vi "trace_display.vi"(0 "Carrier amplitudes":T13 format="%#_3p", 1 "Ref carrier amplitudes":T13 format="%#_3p", 2 "Frequency display":T12, 3 "Spectrogram reference":refnum<vi>, 9 "Config":T19={"IO params"={"Conversion"={"Rate"=4.0, "In cards"=2, "Out channels"=4}, "Carriers"={"Phase shift"=180.0, "Levels"=[[0.8, 0.8, 0.8], [0.03, 0.03, 0.03]], "Delay samples"=73.15}}, "High rate STFT"={"Win param"=101.5, "Window type"=61, "Win order"=2, "DFT size"=64, "Channels"=[7], "Oversample"=64}, "Low rate STFT"={"Win param"=120.0, "Window type"=61, "Win order"=8, "DFT size"=64, "Channels"=[7], "Oversample"=64}, "Filtering"={"Hum"={"Frequency"=0.0, "Tc"=0.0, "Limit"=101.5, "FFT filter"=FALSE, "Detrend mode"=enum."Robust linear", "Enable"=FALSE}, "Kalman"={"Process noise"=101.5, "Measure noise"=101.5}, "Distortion"={"LF cut"=101.5, "Tc"=3.0, "Limit"=101.5, "FFT filter"=FALSE, "Detrend mode"=enum."Robust linear", "Enable"=FALSE}}} {"Filtering"."Distortion"."Limit" format="%#_3p"; "Filtering"."Distortion"."LF cut" format="%#_3p"; "Filtering"."Kalman"."Measure noise" format="%#_3p"; "Filtering"."Kalman"."Process noise" format="%#_3p"; "Filtering"."Hum"."Limit" format="%#_3p"; "Filtering"."Hum"."Frequency" format="%#_4p"; "Low rate STFT"."Oversample" min=1 step=1; "Low rate STFT"."Channels" min=0 step=1; "Low rate STFT"."DFT size" min=1 step=1; "Low rate STFT"."Window type" items=["Rectangle"=0, "Hanning"=1, "Hamming"=2, "Blackman-Harris"=3, "Exact Blackman"=4, "Blackman"=5, "Flat Top"=6, "4 Term B-Harris "=7, "7 Term B-Harris"=8, "Low Sidelobe"=9, "Blackman Nuttall"=11, "Triangle"=30, "Bartlett-Hanning"=31, "Bohman"=32, "Parzen"=33, "Welch"=34, "Kaiser"=60, "Dolph-Chebyshev"=61, "Gaussian"=62]; "High rate STFT"."Oversample" min=1 step=1; "High rate STFT"."Channels" min=0 step=1; "High rate STFT"."DFT size" min=1 step=1; "High rate STFT"."Window type" items=["Rectangle"=0, "Hanning"=1, "Hamming"=2, "Blackman-Harris"=3, "Exact Blackman"=4, "Blackman"=5, "Flat Top"=6, "4 Term B-Harris "=7, "7 Term B-Harris"=8, "Low Sidelobe"=9, "Blackman Nuttall"=11, "Triangle"=30, "Bartlett-Hanning"=31, "Bohman"=32, "Parzen"=33, "Welch"=34, "Kaiser"=60, "Dolph-Chebyshev"=61, "Gaussian"=62]; "IO params"."Carriers"."Levels" min=0.0 step=0.1; "IO params"."Conversion"."Rate" format="%#_8g"}, 10 "Reset":bool, 11 "Modulation info":T18 {"Hi channels at low" min=0 step=1; "Low carriers" format="%#_6p"; "High carriers" format="%#_6p"}, 12 "Display options":T3={"Display card"=0, "Signal"=enum."Raw data", "Source axis"=enum."X", "Sensor axis"=enum."X", "Spectrum parameters"={"Window"=enum."7 Term B-Harris", "FFT blocking"=enum."1", "Averaging"=5.0, "Order"=2}, "AC/DC"=enum."Radio Selection 1", "Levels selectors"=[], "Map selector"=enum."fire", "Restart Averaging"=FALSE, "Noise ref"=FALSE} {"Spectrum parameters"."Order" min=1 max=100; "Spectrum parameters"."Averaging" min=0.0 max=1000.0 step=1.0}, 13 "Trace info":T15) -> (20 "Autocorrelation":T1, 21 "Levels arrays":cluster{"Levels":dbl[][]}[](array[cluster]), 22 "STFT Spectrogram":dbl[][](array[numeric]), 23 "Time domain":waveform(dbl)[](array[waveform]), 24 "Time statistics":T14 {"dB" format="%.1f"; "RMS" format="%#_3p"; "DC" format="%#_3p"; "|max|" format="%#_3p"}, 25 "Spectrum":waveform(dbl)[](array[waveform]), 26 "Noise":T2 {"Noise delta" format="%#_6p"; "Noise floor" format="%#_6p"})   [LabVIEW 2014]
uses:
  ilemt_config.ctl
  IO_params.ctl
  stft_params.ctl
  <vilib>/Analysis/4window.llb/windowTd.ctl
  filter_params.ctl
  detrend_mode.ctl
  modulation_info.ctl
  trace_info.ctl
  trace_channel.ctl
  ilemt_status.ctl
  carrier_amplitudes.ctl
  trace_stats.ctl
  frequency_display_tabs.ctl
  display_options.ctl
  display_source.ctl
  axis_name.ctl
  spectrum_parameters.ctl
  levels_selector.ctl
  Level selector 1.ctl
  Level selector 4.ctl
  Level selector 3.ctl
  Level selector 2.ctl
  <vilib>/Analysis/2dsp.llb/Inverse Real FFT.vi
  <vilib>/Analysis/2dsp.llb/1D Auto Correlation (DBL).vi
  <vilib>/Analysis/NI_AALPro.lvlib
panel:
  in  "Autocorrelation normalization":enum32{"none", "unbiased", "biased"}(ring)=enum."biased"
  # "Options:"
  # "High"
  # "Low"
  # "X"
  # "Y"
  # "Z"
  # "High"
  # "Low"
  # "X"
  # "Y"
  # "Z"
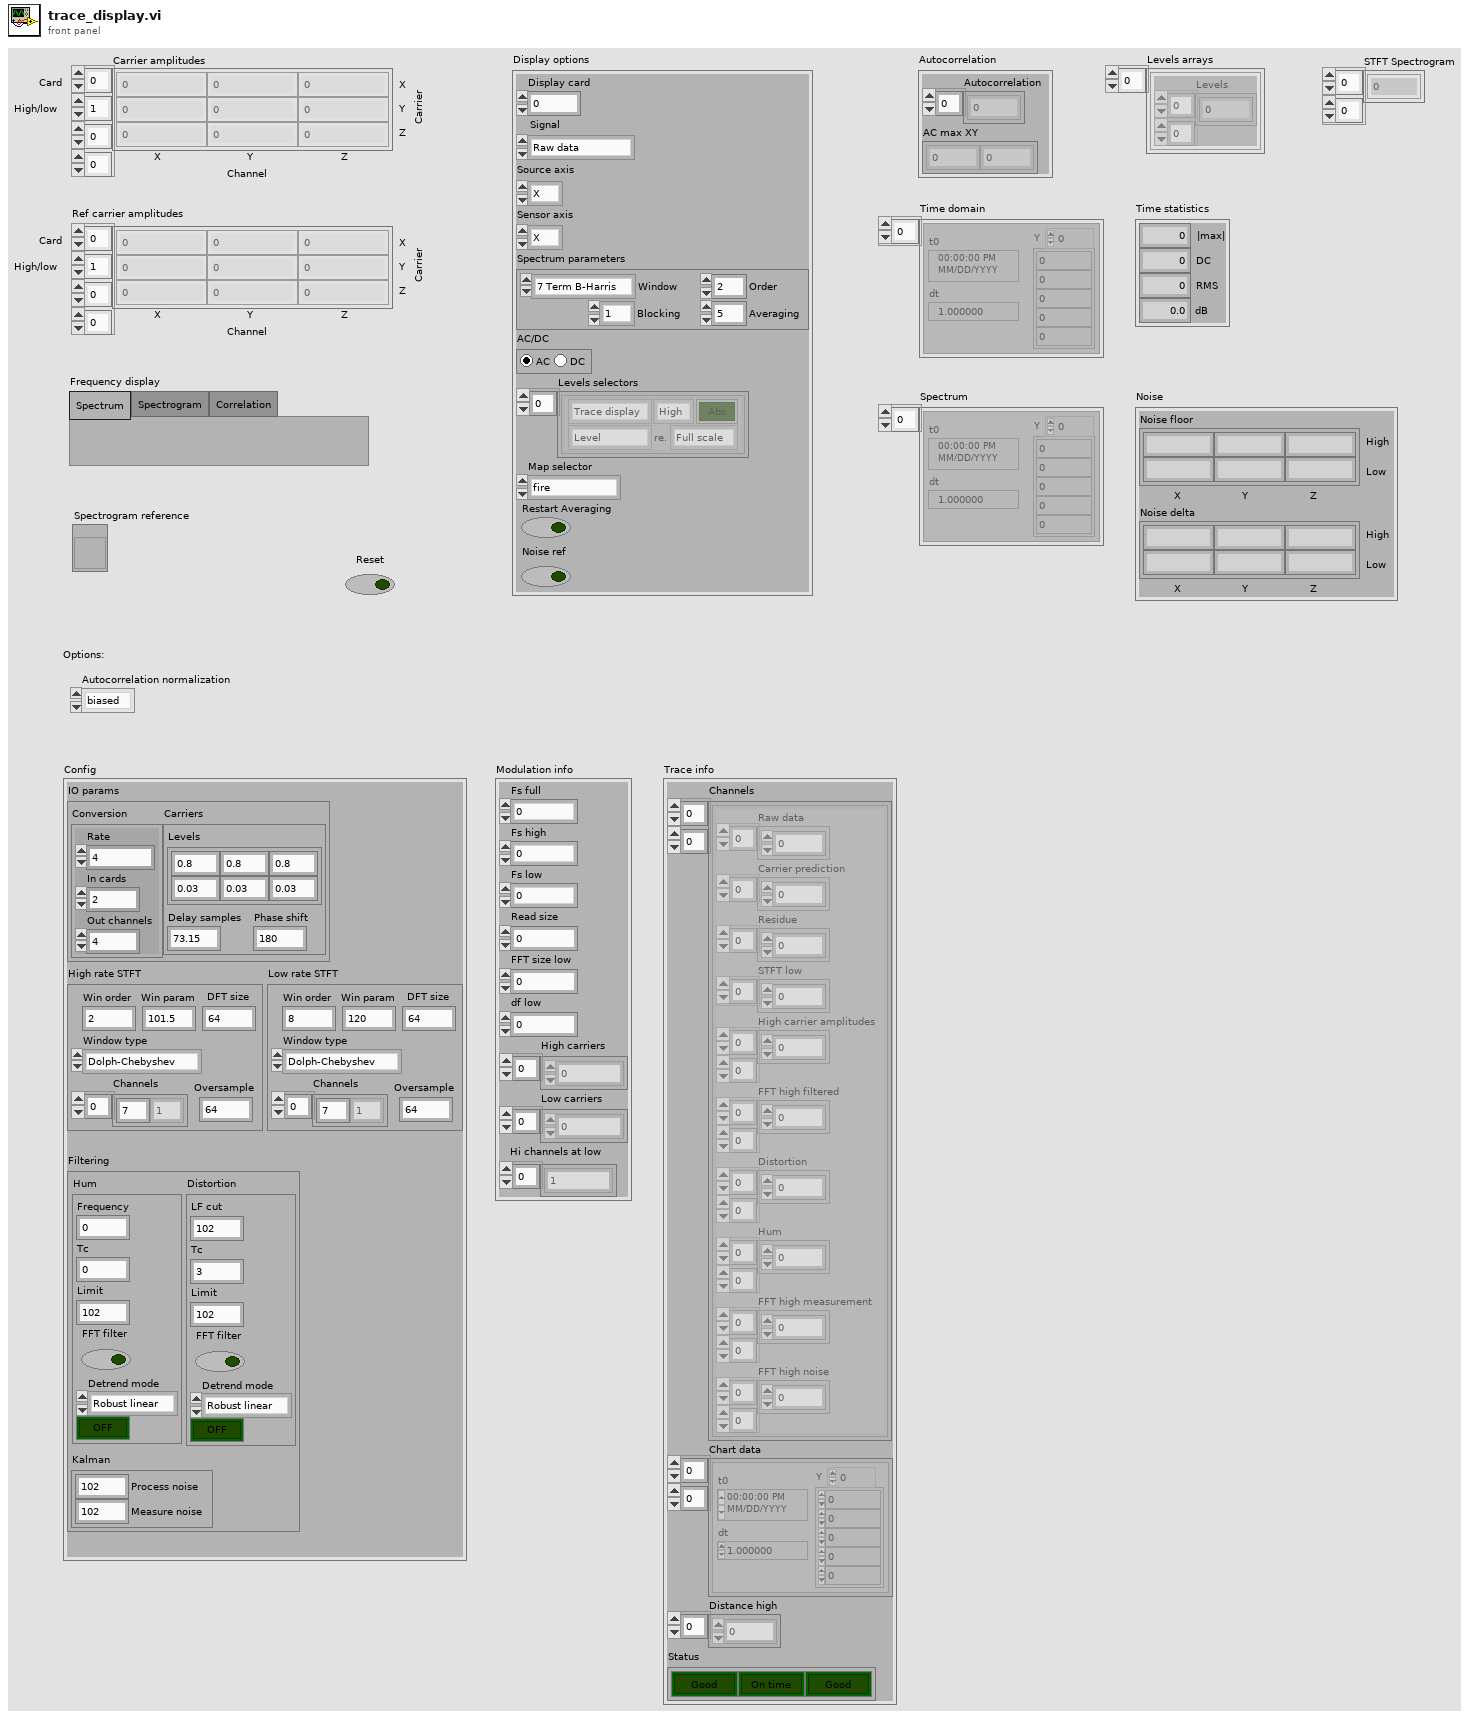
[diagram p1: front panel]
types:
  T1 = cluster{"Autocorrelation":dbl[], "AC max XY":dbl[]}
  T2 = cluster{"Noise floor":dbl[][], "Noise delta":dbl[][]}
  T3 = typedef "display_options.ctl" = cluster{"Display card":i32, "Signal":T4, "Source axis":T5, "Sensor axis":T5, "Spectrum parameters":T6, "AC/DC":enum32{"Radio Selection 1", "Radio Selection 2"}, "Levels selectors":T7[], "Map selector":enum16{"fire", "rainbow", "grey", "inverse grey", "ice", "original"}, "Restart Averaging":bool, "Noise ref":bool}
  T4 = typedef "display_source.ctl" = enum16{"Raw data", "Carrier predict", "Residue", "STFT low", "Hum amplitude", "Hum phase", "Distortion amplitude", "Distortion phase", "FFT high noise", "FFT high measurement", "FFT high filtered", "Amplitude high", "Distance high", "Chart high", "Chart low"}
  T5 = typedef "axis_name.ctl" = enum16{"X", "Y", "Z"}
  T6 = typedef "spectrum_parameters.ctl" = cluster{"Window":enum16{"None ", "Hanning", "Hamming", "Blackman-Harris", "Exact Blackman", "Blackman", "Flat Top", "4 Term B-Harris ", "7 Term B-Harris", "Low Sidelobe"}, "FFT blocking":enum16{"1", "2", "4", "8"}, "Averaging":dbl, "Order":u32}
  T7 = typedef "levels_selector.ctl" = cluster{"Signal source":T8, "Mode":T9, "re.":T10, "High/low":T11, "Sense":bool}
  T8 = typedef "Level selector 1.ctl" = enum16{"Trace display", "Carrier levels", "Ref levels", "Distortion"}
  T9 = typedef "Level selector 4.ctl" = enum16{"Level", "dB", "Phase", "Mismatch"}
  T10 = typedef "Level selector 3.ctl" = enum16{"Full scale", "Carrier", "Ref level", "Noise"}
  T11 = typedef "Level selector 2.ctl" = enum16{"High", "Low"}
  T12 = typedef "frequency_display_tabs.ctl" = enum32{"Spectrum", "Spectrogram", "Correlation"}
  T13 = typedef "carrier_amplitudes.ctl" = cdb[][][][]
  T14 = typedef "trace_stats.ctl" = cluster{"|max|":dbl, "DC":dbl, "RMS":dbl, "dB":dbl}
  T15 = typedef "trace_info.ctl" = cluster{"Channels":T16[][], "Chart data":waveform(dbl)[][], "Distance high":dbl[], "Status":T17}
  T16 = typedef "trace_channel.ctl" = cluster{"Raw data":dbl[], "Carrier prediction":dbl[], "Residue":dbl[], "STFT low":cdb[], "High carrier amplitudes":cdb[][], "FFT high filtered":cdb[][], "Distortion":cdb[][], "Hum":cdb[][], "FFT high measurement":cdb[][], "FFT high noise":dbl[][]}
  T17 = typedef "ilemt_status.ctl" = cluster{"NaN":bool, "Backlog":bool, "Clipping":bool}
  T18 = typedef "modulation_info.ctl" = cluster{"Fs full":dbl, "Fs high":dbl, "Fs low":dbl, "Read size":i32, "FFT size low":i32, "df low":dbl, "High carriers":dbl[], "Low carriers":dbl[], "Hi channels at low":i32[]}
  T19 = typedef "ilemt_config.ctl" = cluster{"IO params":T20, "High rate STFT":T21, "Low rate STFT":T21, "Filtering":T23}
  T20 = typedef "IO_params.ctl" = cluster{"Conversion":cluster{"Rate":dbl, "In cards":u32, "Out channels":u32}, "Carriers":cluster{"Phase shift":dbl, "Levels":dbl[][], "Delay samples":dbl}}
  T21 = typedef "stft_params.ctl" = cluster{"Win param":dbl, "Window type":T22, "Win order":i32, "DFT size":i32, "Channels":i32[], "Oversample":i32}
  T22 = typedef "NI_AALPro.lvlib/windowTd.ctl" = u32
  T23 = typedef "filter_params.ctl" = cluster{"Hum":cluster{"Frequency":dbl, "Tc":dbl, "Limit":dbl, "FFT filter":bool, "Detrend mode":T24, "Enable":bool}, "Kalman":cluster{"Process noise":dbl, "Measure noise":dbl}, "Distortion":cluster{"LF cut":dbl, "Tc":dbl, "Limit":dbl, "FFT filter":bool, "Detrend mode":T24, "Enable":bool}}
  T24 = typedef "detrend_mode.ctl" = enum16{"Zero mean", "Linear", "Robust linear"}
  T25 = enum16{"fire", "rainbow", "grey", "inverse grey", "ice", "original"}
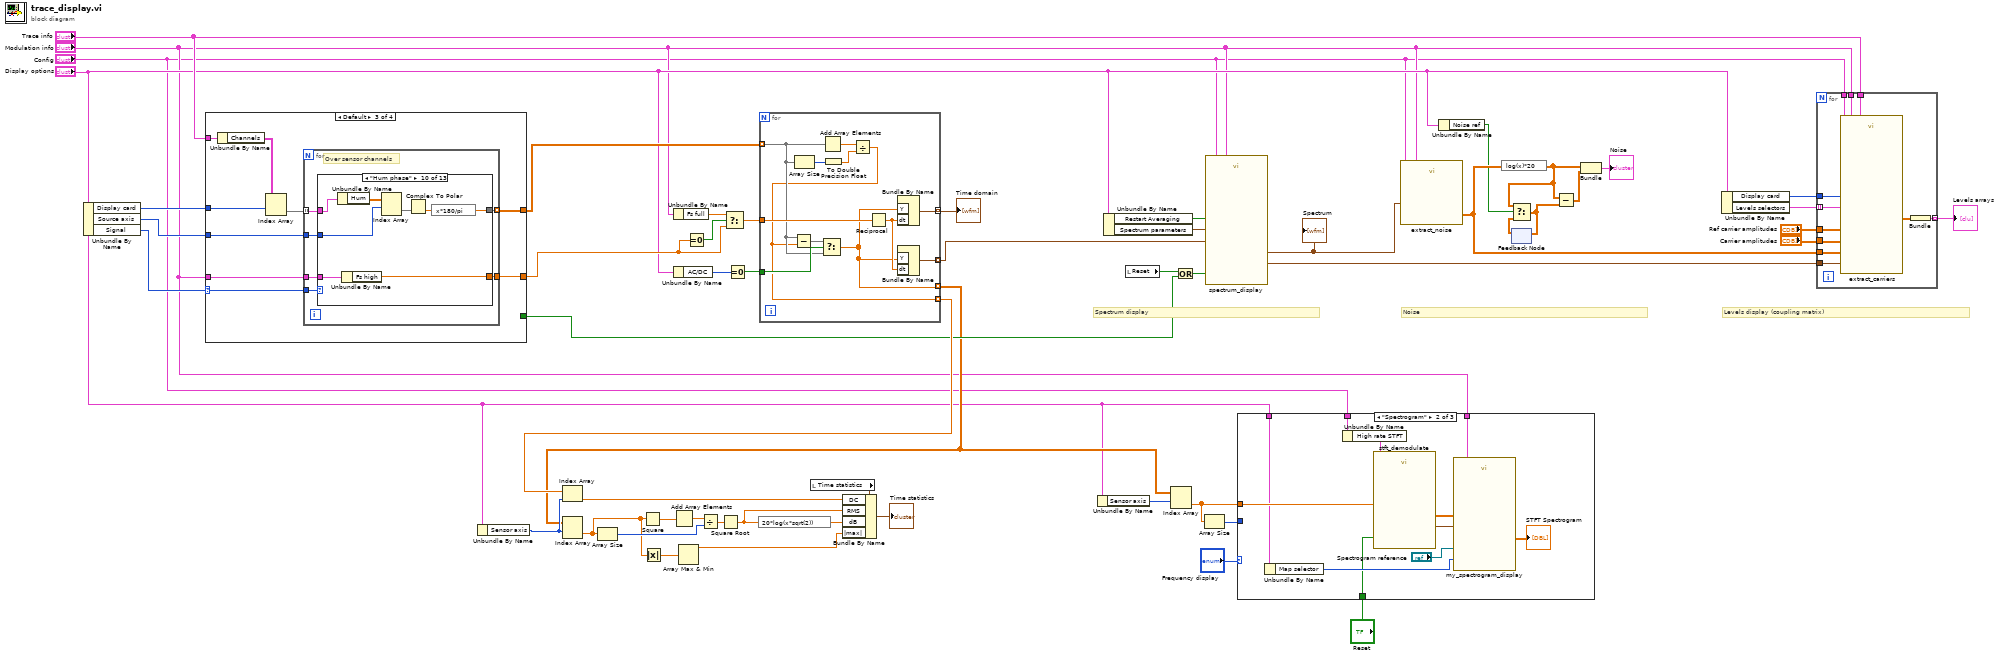
[diagram p0: block diagram]
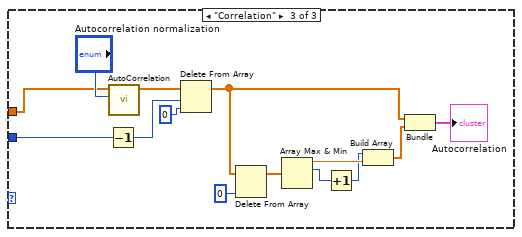
[diagram p3: hidden frame]
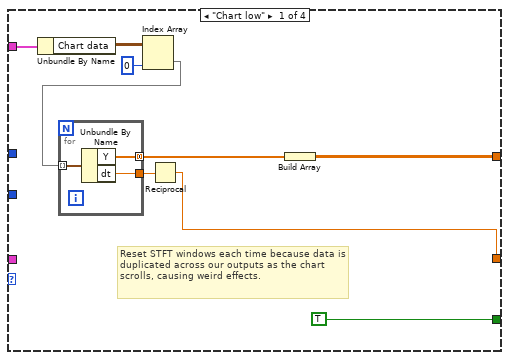
[diagram p4: hidden frame]
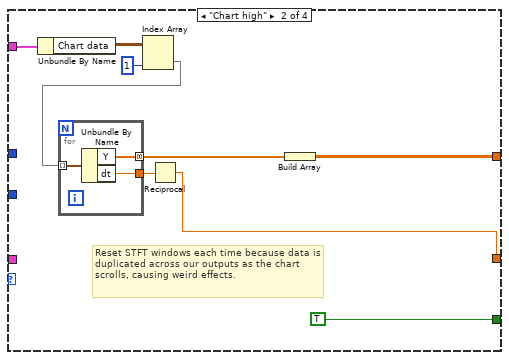
[diagram p5: hidden frame]
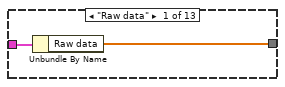
[diagram p6: hidden frame]
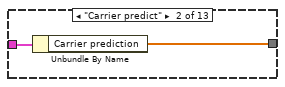
[diagram p7: hidden frame]
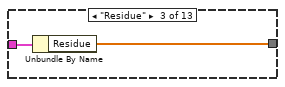
[diagram p8: hidden frame]
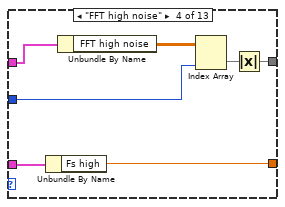
[diagram p9: hidden frame]
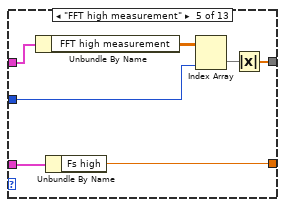
[diagram p10: hidden frame]
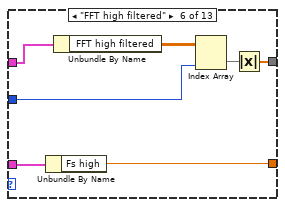
[diagram p11: hidden frame]
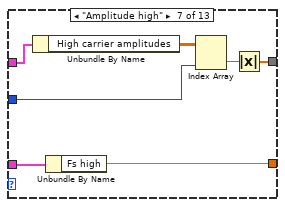
[diagram p12: hidden frame]
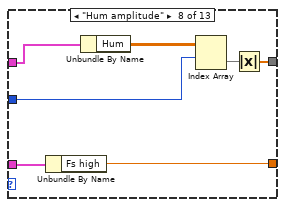
[diagram p13: hidden frame]
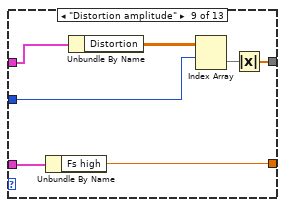
[diagram p14: hidden frame]
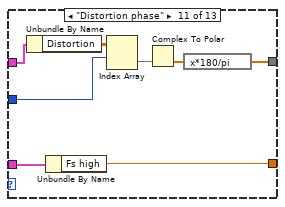
[diagram p15: hidden frame]
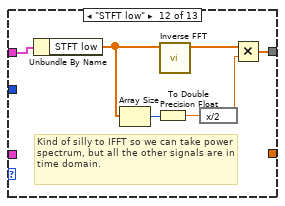
[diagram p16: hidden frame]
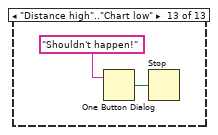
[diagram p17: hidden frame]
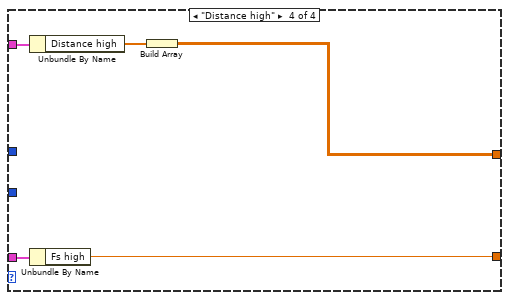
[diagram p18: hidden frame]
diagram:
  # "Levels display (coupling matrix)"
  # "Noise"
  # "Spectrum display"
  n1 = Unbundle By Name("Display options") -> ("Display card"=w25:i32, "Source axis"=w24:T5, "Signal"=w23:T4)
  n2 = case shown="Default" w23 {
    selector: w23 -> [_ _ w84 _]
    tunnel: "Trace info" -> [w60 w72 w85 w170]
    tunnel: [w57 w69 w88 w168] -> w38
    tunnel: "Modulation info" -> [_ _ w87 w172]
    tunnel: [w59 w71 w86 w171] -> w12
    tunnel: [TRUE TRUE _ _] -> w29
    tunnel: w24 -> [_ _ w83 _]
    tunnel: w25 -> [_ _ w80 _]
    frame "Chart low" {
      # "Reset STFT windows each time because data is duplicated across our outputs as the chart scrolls, causing weird effects."
      n3 = Unbundle By Name(w60) -> ("Chart data"=w64:waveform(dbl)[][])
      n4 = Index Array(array=w64, index (col)=0 ("index (row)")) -> (element=w63:waveform(dbl)[])  [unwired: 1 in]
      n5 = for {
        tunnel: w63 -> [w67] mode=indexing
        tunnel: [w66] -> w58 mode=concatenating
        tunnel: [w65] -> w61
        n6 = Unbundle By Name(w67) -> ("Y"=w66:dbl[], "dt"=w65:dbl)
      }
      n7 = Reciprocal(x=w61) -> (1/x=w59:dbl)
      n8 = Build Array(w58) -> (w57:dbl[][])
    }
    frame "Chart high" {
      # "Reset STFT windows each time because data is duplicated across our outputs as the chart scrolls, causing weird effects."
      n9 = Unbundle By Name(w72) -> ("Chart data"=w76:waveform(dbl)[][])
      n10 = Index Array(array=w76, index (col)=1 ("index (row)")) -> (element=w75:waveform(dbl)[])  [unwired: 1 in]
      n11 = for {
        tunnel: w75 -> [w79] mode=indexing
        tunnel: [w78] -> w70 mode=concatenating
        tunnel: [w77] -> w73
        n12 = Unbundle By Name(w79) -> ("Y"=w78:dbl[], "dt"=w77:dbl)
      }
      n13 = Reciprocal(x=w73) -> (1/x=w71:dbl)
      n14 = Build Array(w70) -> (w69:dbl[][])
    }
    frame Default {
      n15 = Unbundle By Name(w85) -> ("Channels"=w82:T16[][])
      n16 = Index Array(array=w82, index (row)=w80) -> (element=w81:T16[])  [unwired: 1 in]
      n17 = for {
        tunnel: [w94] -> w88 mode=indexing
        tunnel: w87 -> [w93]
        tunnel: [w92] -> w86
        tunnel: w84 -> [w91]
        tunnel: w81 -> [w90] mode=indexing
        tunnel: w83 -> [w89]
        # "Over sensor channels"
        n18 = case shown="\"Hum phase\"" w91 {
          tunnel: w90 -> [w96 w98 w100 w107 w114 w121 w128 w135 w142 w150 w158 w165 _]
          tunnel: [w95 w97 w99 w102 w109 w116 w123 w130 w137 w143 w151 w161 _] -> w94
          tunnel: [_ _ _ w105 w112 w119 w126 w133 w140 w148 w156 _ _] -> w92
          tunnel: w93 -> [_ _ _ w106 w113 w120 w127 w134 w141 w149 w157 _ _]
          tunnel: w89 -> [_ _ _ w101 w108 w115 w122 w129 w136 w146 w154 _ _]
          frame "Raw data" {
            n19 = Unbundle By Name(w96) -> ("Raw data"=w95:dbl[])
          }
          frame "Carrier predict" {
            n20 = Unbundle By Name(w98) -> ("Carrier prediction"=w97:dbl[])
          }
          frame "Residue" {
            n21 = Unbundle By Name(w100) -> ("Residue"=w99:dbl[])
          }
          frame "FFT high noise" {
            n22 = Unbundle By Name(w106) -> ("Fs high"=w105:dbl)
            n23 = Unbundle By Name(w107) -> ("FFT high noise"=w104:dbl[][])
            n24 = Index Array(array=w104, index (col)=w101) -> (element=w103:dbl[])  [unwired: 1 in]
            n25 = Absolute Value(x=w103) -> (abs(x)=w102:dbl[])
          }
          frame "FFT high measurement" {
            n26 = Unbundle By Name(w114) -> ("FFT high measurement"=w111:cdb[][])
            n27 = Unbundle By Name(w113) -> ("Fs high"=w112:dbl)
            n28 = Index Array(array=w111, index (col)=w108) -> (element=w110:cdb[])  [unwired: 1 in]
            n29 = Absolute Value(x=w110) -> (abs(x)=w109:dbl[])
          }
          frame "FFT high filtered" {
            n30 = Unbundle By Name(w120) -> ("Fs high"=w119:dbl)
            n31 = Unbundle By Name(w121) -> ("FFT high filtered"=w118:cdb[][])
            n32 = Index Array(array=w118, index (col)=w115) -> (element=w117:cdb[])  [unwired: 1 in]
            n33 = Absolute Value(x=w117) -> (abs(x)=w116:dbl[])
          }
          frame "Amplitude high" {
            n34 = Unbundle By Name(w128) -> ("High carrier amplitudes"=w125:cdb[][])
            n35 = Unbundle By Name(w127) -> ("Fs high"=w126:dbl)
            n36 = Index Array(array=w125, index (col)=w122) -> (element=w124:cdb[])  [unwired: 1 in]
            n37 = Absolute Value(x=w124) -> (abs(x)=w123:dbl[])
          }
          frame "Hum amplitude" {
            n38 = Unbundle By Name(w134) -> ("Fs high"=w133:dbl)
            n39 = Unbundle By Name(w135) -> ("Hum"=w132:cdb[][])
            n40 = Index Array(array=w132, index (row)=w129) -> (element=w131:cdb[])  [unwired: 1 in]
            n41 = Absolute Value(x=w131) -> (abs(x)=w130:dbl[])
          }
          frame "Distortion amplitude" {
            n42 = Unbundle By Name(w141) -> ("Fs high"=w140:dbl)
            n43 = Unbundle By Name(w142) -> ("Distortion"=w139:cdb[][])
            n44 = Index Array(array=w139, index (row)=w136) -> (element=w138:cdb[])  [unwired: 1 in]
            n45 = Absolute Value(x=w138) -> (abs(x)=w137:dbl[])
          }
          frame "Hum phase" {
            n46 = Unbundle By Name(w150) -> ("Hum"=w147:cdb[][])
            n47 = Unbundle By Name(w149) -> ("Fs high"=w148:dbl)
            n48 = Index Array(array=w147, index (row)=w146) -> (element=w145:cdb[])  [unwired: 1 in]
            n49 = Complex To Polar(r * e^(i*theta)=w145) -> (theta=w144:dbl[])  [unwired: 1 out]
            n50 = expression code="x*180/pi"(w144) -> (w143:dbl[])
          }
          frame "Distortion phase" {
            n51 = Unbundle By Name(w158) -> ("Distortion"=w155:cdb[][])
            n52 = Unbundle By Name(w157) -> ("Fs high"=w156:dbl)
            n53 = Index Array(array=w155, index (row)=w154) -> (element=w153:cdb[])  [unwired: 1 in]
            n54 = Complex To Polar(r * e^(i*theta)=w153) -> (theta=w152:dbl[])  [unwired: 1 out]
            n55 = expression code="x*180/pi"(w152) -> (w151:dbl[])
          }
          frame "STFT low" {
            # "Kind of silly to IFFT so we can take power spectrum, but all the other signals are in time domain."
            n56 = Unbundle By Name(w165) -> ("STFT low"=w159:cdb[])
            n57 = Array Size(array=w159) -> (size(s)=w163:i32)
            n58 = To Double Precision Float(number=w163) -> (double precision float=w164:dbl)
            n59 = call-poly <vilib>:"Inverse FFT.vi"("FFT {X}"=w159) -> ("X"=w162:dbl[])  [unwired: 9 in, 1 out]
            n60 = expression code="x/2"(w164) -> (w160:dbl)
            n61 = Multiply(x=w162, y=w160) -> (x*y=w161:dbl[])
          }
          frame "Distance high".."Chart low" {
            n62 = One Button Dialog(message="Shouldn't happen!") -> (true=w167:bool)  [unwired: 1 in]
            n63 = Stop(stop? (T)=w167) -> ()
          }
        }
      }
    }
    frame "Distance high" {
      n64 = Unbundle By Name(w170) -> ("Distance high"=w169:dbl[])
      n65 = Unbundle By Name(w172) -> ("Fs high"=w171:dbl)
      n66 = Build Array(w169) -> (w168:dbl[][])
    }
  }
  n67 = Unbundle By Name("Display options") -> ("Sensor axis"=w11:T5)
  n68 = Unbundle By Name("Modulation info") -> ("Fs full"=w45:dbl)
  n69 = Unbundle By Name("Display options") -> ("AC/DC"=w16:enum32{"Radio Selection 1", "Radio Selection 2"})
  n70 = Equal To 0?(x=w12) -> (x = 0?=w44:bool)
  n71 = Select(t=w45, s=w44, f=w12) -> (s? t:f=w43:dbl)
  n72 = Equal To 0?(x=w16) -> (x = 0?=w26:bool)
  n73 = for {
    tunnel: [w183] -> w42 mode=indexing
    tunnel: [w174] -> w40 mode=indexing
    tunnel: [w173] -> w9 mode=indexing
    tunnel: w43 -> [w180]
    tunnel: [w178] -> w41 mode=indexing
    tunnel: w38 -> [w175] mode=indexing
    tunnel: w26 -> [w176]
    n74 = Array Size(array=w175) -> (size(s)=w184:i32)
    n75 = Add Array Elements(numeric array=w175) -> (sum=w182:dbl)
    n76 = To Double Precision Float(number=w184) -> (double precision float=w181:dbl)
    n77 = Divide(x=w182, y=w181) -> (x/y=w174:dbl)
    n78 = Subtract(x=w175, y=w174) -> (x-y=w177:dbl[])
    n79 = Select(t=w177, s=w176, f=w175) -> (s? t:f=w173:dbl[])
    n80 = Reciprocal(x=w180) -> (1/x=w179:dbl)
    n81 = Bundle By Name("Y"=w173, "dt"=w179) -> (w183:waveform(dbl))  [unwired: 1 in]
    n82 = Bundle By Name("Y"=w173, "dt"=w179) -> (w178:waveform(dbl))  [unwired: 1 in]
  }
  "Time domain" <- w42
  n83 = Index Array(array=w40, index=w11) -> (element=w39:dbl)
  n84 = Index Array(array=w9, index (row)=w11) -> (element=w35:dbl[])  [unwired: 1 in]
  n85 = Array Size(array=w35) -> (size(s)=w52:i32)
  n86 = Square(x=w35) -> (x^2=w55:dbl[])
  n87 = Absolute Value(x=w35) -> (abs(x)=w50:dbl[])
  n88 = Add Array Elements(numeric array=w55) -> (sum=w54:dbl)
  n89 = Array Max & Min(array=w50) -> (max value=w49:dbl)  [unwired: 3 out]
  n90 = Divide(x=w54, y=w52) -> (x/y=w53:dbl)
  n91 = Square Root(x=w53) -> (sqrt(x)=w46:dbl)
  n92 = expression code="20*log(x*sqrt(2))"(w46) -> (w47:dbl)
  n93 = local read "Time statistics"() -> (w51:T14)
  n94 = Bundle By Name(cluster=w51, "DC"=w39, "RMS"=w46, "dB"=w47, "|max|"=w49) -> (→"Time statistics":T14)
  n95 = Unbundle By Name("Display options") -> ("Sensor axis"=w10:T5)
  n96 = Unbundle By Name("Display options") -> ("Restart Averaging"=w18:bool, "Spectrum parameters"=w17:T6)
  n97 = local read "Reset"() -> (w1:bool)
  n98 = Index Array(array=w9, index (row)=w10) -> (element=w8:dbl[])  [unwired: 1 in]
  n99 = Or(x=w1, y=w29) -> (x .or. y?=w28:bool)
  n100 = Array Size(array=w8) -> (size(s)=w7:i32)
  n101 = call "spectrum_display.vi"("Modulation info"="Modulation info", "Reset STFT"=w28, "Config"="Config", "Restart Averaging"=w18, "Spectrum parameters"=w17, "Time domain wavevorms"=w41) -> ("Complex spectrum"=w30:waveform(cdb)[], "dB spectrum"=w31:waveform(dbl)[])  [unwired: 4 in]
  "Spectrum" <- w31
  n102 = case shown="\"Spectrogram\"" "Frequency display" {
    tunnel: w7 -> [_ _ w200]
    tunnel: w8 -> [_ w190 w196]
    tunnel: "Config" -> [_ w189 _]
    tunnel: "Modulation info" -> [_ w188 _]
    tunnel: "Display options" -> [_ w187 _]
    tunnel: "Reset" -> [_ w185 _]
    frame "Spectrum", Default {
    }
    frame "Spectrogram" {
      n103 = Unbundle By Name(w187) -> ("Map selector"=w186:T25)
      n104 = Unbundle By Name(w189) -> ("High rate STFT"=w193:T21)
      n105 = call "stft_demodulate.vi"("STFT params"=w193, "Reset"=w185, "X"=w190) -> ("time-freq sample info"=w192:cluster{"time steps":i32, "frequency bins":i32}, "STFT"=w191:cdb[][])  [unwired: 6 in, 1 out]
      n106 = call "my_spectrogram_display.vi"("Modulation info"=w188, "time-freq sample info"=w192, "Map selector"=w186, "IntensityGraph in"="Spectrogram reference", "STFT {X}"=w191) -> ("STFT Spectrogram"=→"STFT Spectrogram":dbl[][])  [unwired: 6 in]
    }
    frame "Correlation" {
      n107 = Decrement(x=w200) -> (x-1=w209:i32)
      n108 = call-poly <vilib>:"AutoCorrelation.vi"("normalization"="Autocorrelation normalization", "X"=w196) -> ("Rxx"=w201:dbl[])  [unwired: 8 in, 1 out]
      n109 = Delete From Array(array=w201, length=w209, index=0) -> (array with subset deleted=w199:dbl[])  [unwired: 1 out]
      n110 = Delete From Array(array=w199, index=0) -> (array with subset deleted=w205:dbl[])  [unwired: 1 in, 1 out]
      n111 = Array Max & Min(array=w205) -> (max value=w204:dbl, max index (indices)=w203:i32)  [unwired: 2 out]
      n112 = Increment(x=w203) -> (x+1=w202:i32)
      n113 = Build Array(w202, w204) -> (w198:dbl[])
      n114 = Bundle("Rxx"=w199, w198) -> (→"Autocorrelation":cluster{"Rxx":dbl[], dbl[]})  [unwired: 1 in]
    }
  }
  n115 = call "extract_noise.vi"("Config"="Config", "Modulation info"="Modulation info", "Spectrum"=w31) -> ("Noise floor"=w34:dbl[][])  [unwired: 8 in]
  n116 = Unbundle By Name("Display options") -> ("Noise ref"=w22:bool)
  n117 = expression code="log(x)*20"(w34) -> (w21:dbl[][])
  n118 = feedback #1() -> (w33:dbl[][])  [unwired: 1 in]
  n119 = Select(t=w21, s=w22, f=w33) -> (s? t:f=w32:dbl[][])
  n120 = feedback-in #1(w32) -> ()
  n121 = Subtract(x=w21, y=w32) -> (x-y=w20:dbl[][])
  n122 = Bundle("Noise floor"=w21, w20) -> (→"Noise":cluster{"Noise floor":dbl[][], dbl[][]})  [unwired: 1 in]
  n123 = Unbundle By Name("Display options") -> ("Display card"=w5:i32, "Levels selectors"=w15:T7[])
  n124 = for {
    tunnel: w30 -> [w220]
    tunnel: "Modulation info" -> [w219]
    tunnel: "Config" -> [w218]
    tunnel: w15 -> [w217] mode=indexing
    tunnel: [w215] -> w37 mode=indexing
    tunnel: w34 -> [w214]
    tunnel: "Trace info" -> [w213]
    tunnel: "Ref carrier amplitudes" -> [w212]
    tunnel: "Carrier amplitudes" -> [w211]
    tunnel: w5 -> [w210]
    n125 = call "extract_carriers.vi"("Carrier amplitudes"=w211, "Config"=w218, "Modulation info"=w219, "Ref carrier amplitudes"=w212, "Display card"=w210, "Level selector"=w217, "Spectrum"=w220, "Trace info"=w213, "Noise floor"=w214) -> ("Levels"=w216:dbl[][])  [unwired: 10 in]
    n126 = Bundle("Levels"=w216) -> (w215:cluster{"Levels":dbl[][]})  [unwired: 1 in]
  }
  "Levels arrays" <- w37
